vi "Home.vi"(8 "error in (no error)":errorcluster, 11 "XYStage in":refnum<class "XYStage.lvclass">) -> (0 "error out":errorcluster, 3 "XYStage out":refnum<class "XYStage.lvclass">)   [LabVIEW 2017, in "XYStage.lvclass"]
uses:
  XYStage.lvclass
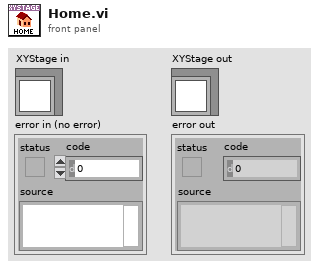
[diagram p1: front panel]
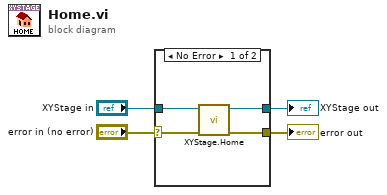
[diagram p0: block diagram]
diagram:
  n1 = case shown="No Error" "error in (no error)" {
    selector: "error in (no error)" -> [w6 w10]
    tunnel: [w5 w10] -> w3
    tunnel: [w7 w9] -> w1
    tunnel: "XYStage in" -> [w8 w9]
    frame No Error {
      n2 = call-dynamic "XYStage.Home.vi"("error in (no error)"=w6, "XYStage in"=w8) -> ("error out"=w5:errorcluster, "XYStage out"=w7:refnum<class "XYStage.lvclass">)  [unwired: 8 in]
    }
    frame Error {
    }
  }
  "error out" <- w3
  "XYStage out" <- w1
